vi "ConnectedAxes.vi"() -> ()   [LabVIEW 2014]
panel:
  out "Connected Axes":string[](array[string])
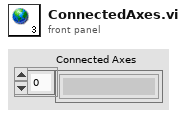
[diagram p1: front panel]
diagram:
